vi "Sequence Read_Write.vi"(7 "Trial or Rig":enum16{"Trial", "Rig"}(ring), 8 "Error IN":errorcluster, 9 "Sequence IN":string[](array[string]), 11 "Select":enum16{"Save Sequence", "Read Sequence"}(ring)) -> (0 "Error OUT":errorcluster, 1 "Sequence OUT":string[](array[string]))   [LabVIEW 2018]
uses:
  Globals/Global - Configuration Options.vi
  <vilib>/Utility/file.llb/Write Delimited Spreadsheet (string).vi
  <vilib>/Utility/file.llb/Read Delimited Spreadsheet (string).vi
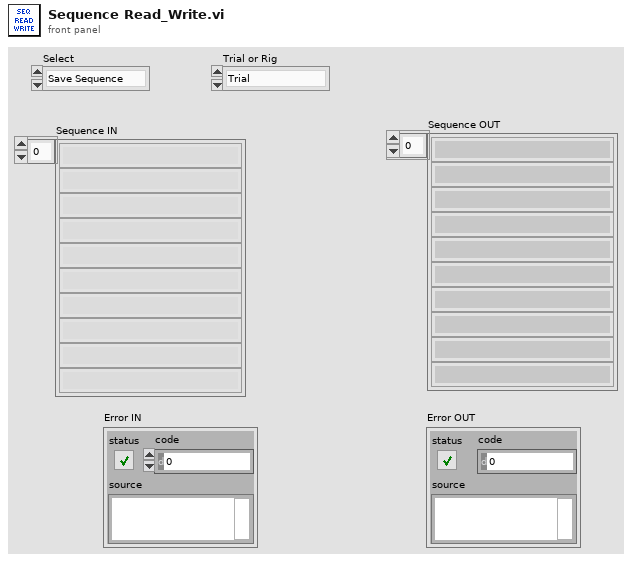
[diagram p1: front panel]
types:
  T1 = typedef "Rig Config Settings.ctl" = cluster{"Rig Name":string, "Rig Room":string, "Base Directory":string, "Computer IP Address":string, "Globals Name":string, "Treatmill Str":string, "cRIO Test Data Dir":path, "ai":string, "ao":string, "dio":string, "A_calib_str_row1":string, "A_calib_str_row2":string, "A_calib_str_row3":string, "Zero_V_str":string, "step_V":string, "Sample Freq":string, "ai_threshold":string, "run_speed_thresh":string, "speed_time_length":string, "wall ball gain":string, "max wall pos":string, "max cor width":string, "Trial Config Directory":path, "Randomize Trials?":bool}
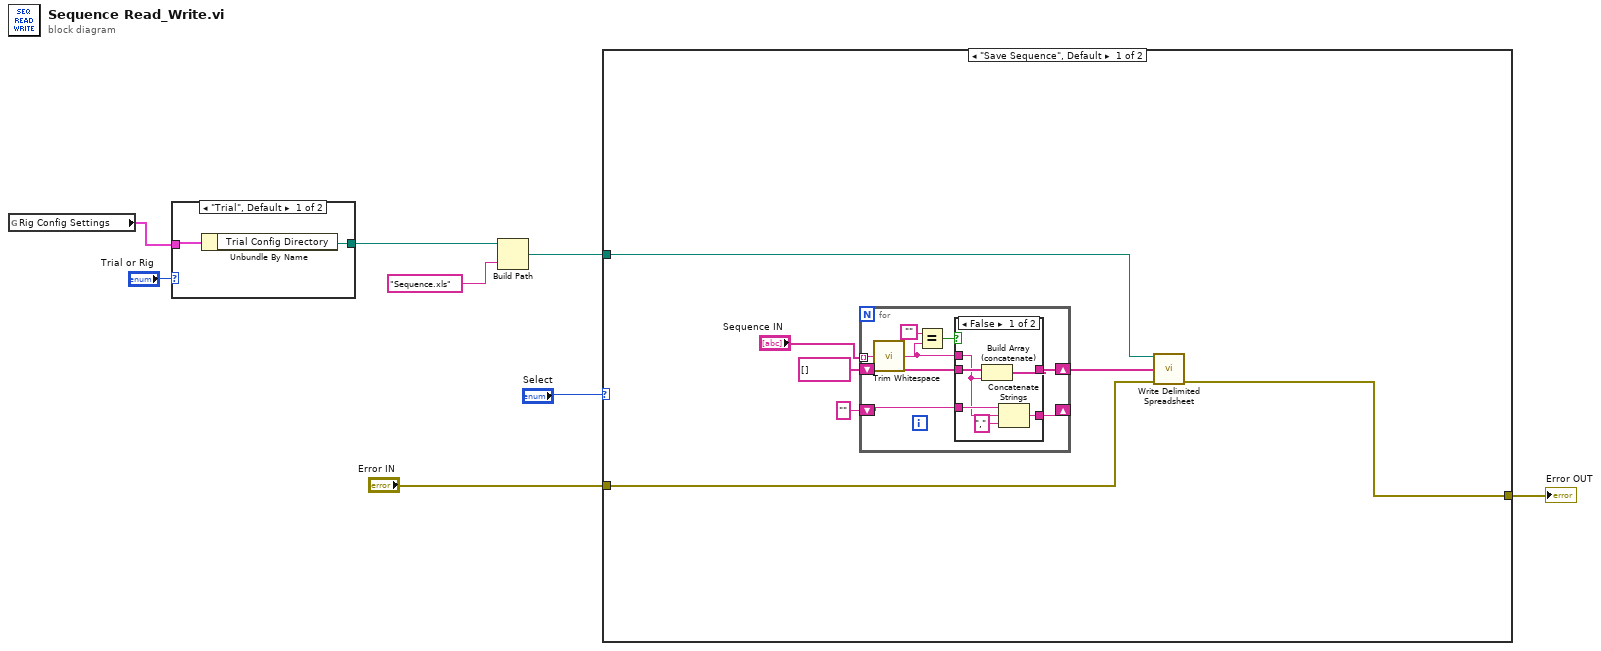
[diagram p0: block diagram]
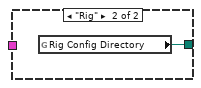
[diagram p2: hidden frame]
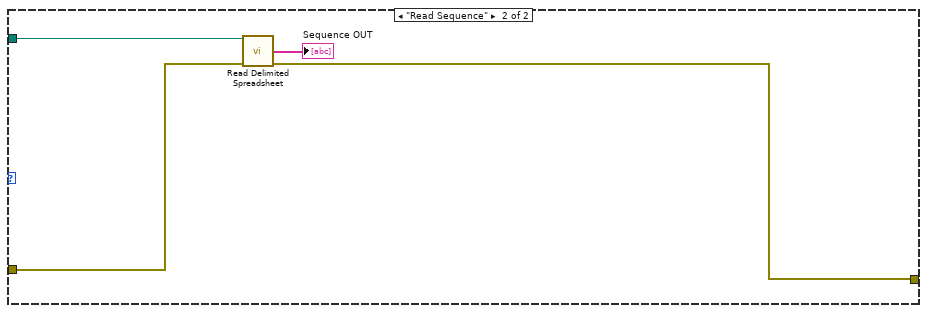
[diagram p4: hidden frame]
diagram:
  n1 = global read "Global - Configuration Options.vi" "Rig Config Settings"() -> (w2:T1)
  n2 = case shown="\"Trial\", Default" "Trial or Rig" {
    tunnel: [w10 w11] -> w5
    tunnel: w2 -> [w9 _]
    frame "Trial", Default {
      n3 = Unbundle By Name(w9) -> ("Trial Config Directory"=w10:path)
    }
    frame "Rig" {
      n4 = global read "Global - Configuration Options.vi" "Rig Config Directory"() -> (w11:path)
    }
  }
  n5 = Build Path(base path=w5, name or relative path="Sequence.xls") -> (appended path=w8:path)
  n6 = case shown="\"Save Sequence\", Default" "Select" {
    tunnel: w8 -> [w18 w38]
    tunnel: [w13 w35] -> w4
    tunnel: "Error IN" -> [w12 w36]
    frame "Save Sequence", Default {
      n7 = for {
        shift-right: [w23] -> w17
        shift-left: string[] [] -> [w24]
        tunnel: "Sequence IN" -> [w22] mode=indexing
        shift-right: [w19] -> _
        shift-left: "" -> [w20]
        n8 = call <vilib>:"Trim Whitespace.vi"("string"=w22) -> ("trimmed string"=w21:string)  [unwired: 1 in]
        n9 = Equal?(x="", y=w21) -> (x = y?=w25:bool)
        n10 = case shown="False" w25 {
          tunnel: w24 -> [w31 w34]
          tunnel: [w32 w34] -> w23
          tunnel: w21 -> [w28 _]
          tunnel: w20 -> [w29 w33]
          tunnel: [w27 w33] -> w19
          frame False {
            n11 = Build Array (concatenate)(w31, w28) -> (w32:string[])
            n12 = Concatenate Strings(w29, w28, "," ("string")) -> (w27:string)
          }
          frame True {
          }
        }
      }
      n13 = call-poly <vilib>:"Write Delimited Spreadsheet.vi"("file path (dialog if empty)"=w18, "1D data"=w17, "error in (no error)"=w12) -> ("error out"=w13:errorcluster)  [unwired: 11 in, 1 out]
    }
    frame "Read Sequence" {
      n14 = call-poly <vilib>:"Read Delimited Spreadsheet.vi"("file path (dialog if empty)"=w38, "error in (no error)"=w36) -> ("first row"=→"Sequence OUT":string[], "error out"=w35:errorcluster)  [unwired: 8 in, 4 out]
    }
  }
  "Error OUT" <- w4
